vi "Main_old.vi"() -> ()   [LabVIEW 2021]
uses:
  TypeDefs/DevInfo.ctl
  TypeDefs/TargetAccess.ctl
  <vilib>/nisyscfg/Network Settings Format.ctl
  <userlib>/S2 Labs/Error Reporting/Transport_WinDebug/Transport_WinDebug.lvclass
  C:/Program Files (x86)/National Instruments/LabVIEW 2021/user.lib/S2 Labs/Error Reporting/Transport Class/Transport.lvclass
  <vilib>/nisyscfg/Close (System).vi
  <vilib>/nisyscfg/Format 5.3.vi
  <vilib>/nisyscfg/Save Changes (Hardware).vi
  <vilib>/nisyscfg/Close (Hardware).vi
  <vilib>/nisyscfg/Save Changes (System).vi
  <vilib>/nisyscfg/nisyscfg.lvlib
  <resource>/objmgr/nisysapi.rc
  <userlib>/S2 Labs/Error Reporting/Error Reporting.lvlib
  <resource>/objmgr/nicontrollersysapi.rc
panel:
  in  "Abort":bool
  out "n":i32
  out "of":i32
  out "Refreshing":bool
  in  "Device List":i32(listbox)
  out "MAC":string
  out "OS":string
  out "Firmware":string
  out "Status":string
  out "Version":string
  out "Description":string
  out "Title":string
  out "Model":string
  in  "ChangePassword":bool
  in  "ChangeMode":bool
  in  "Restart":bool
  in  "FormatDisk":bool
  in  "ManageFeeds":bool
  in  "DeplyFW":bool
  in  "NetworkSettings":bool
  in  "Refresh":bool
  in  "DeplyImg":bool
  in  "RetrieveImg":bool
  # "Device Properties"
  # "Image Properties"
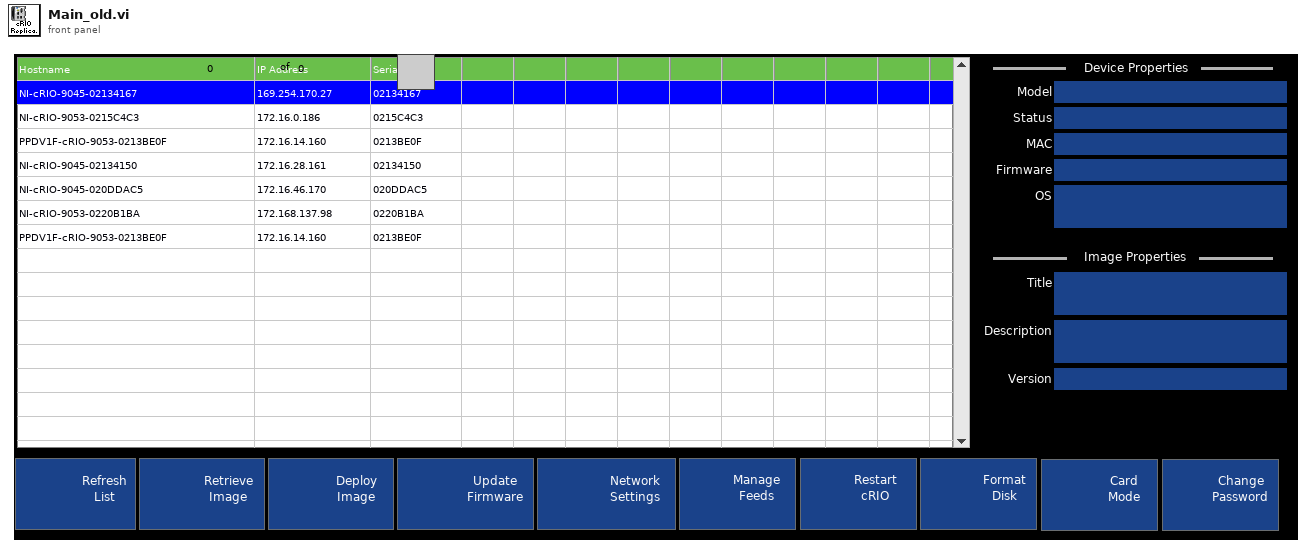
[diagram p1: front panel]
types:
  T1 = typedef "DevInfo.ctl" = cluster{"Hostname":string, "IPAddress":string, "MAC":string, "SerialNum":string, "Model":string, "Status":string, "FW":string, "OSDesc":string, "ImgTitle":string, "ImgDesc":string, "ImgVer":string, "ImgID":string, "IP Address Request Mode":i32, "SubnetMask":string, "Gateway":string, "DNSServer":string}
  T2 = enum8{"Enabled", "Disabled", "Disabled and Grayed Out"}
  T3 = typedef "TargetAccess.ctl" = enum16{"Read-Only", "Admin"}
  T4 = typedef "nisyscfg.lvlib/Network Settings Format.ctl" = u32
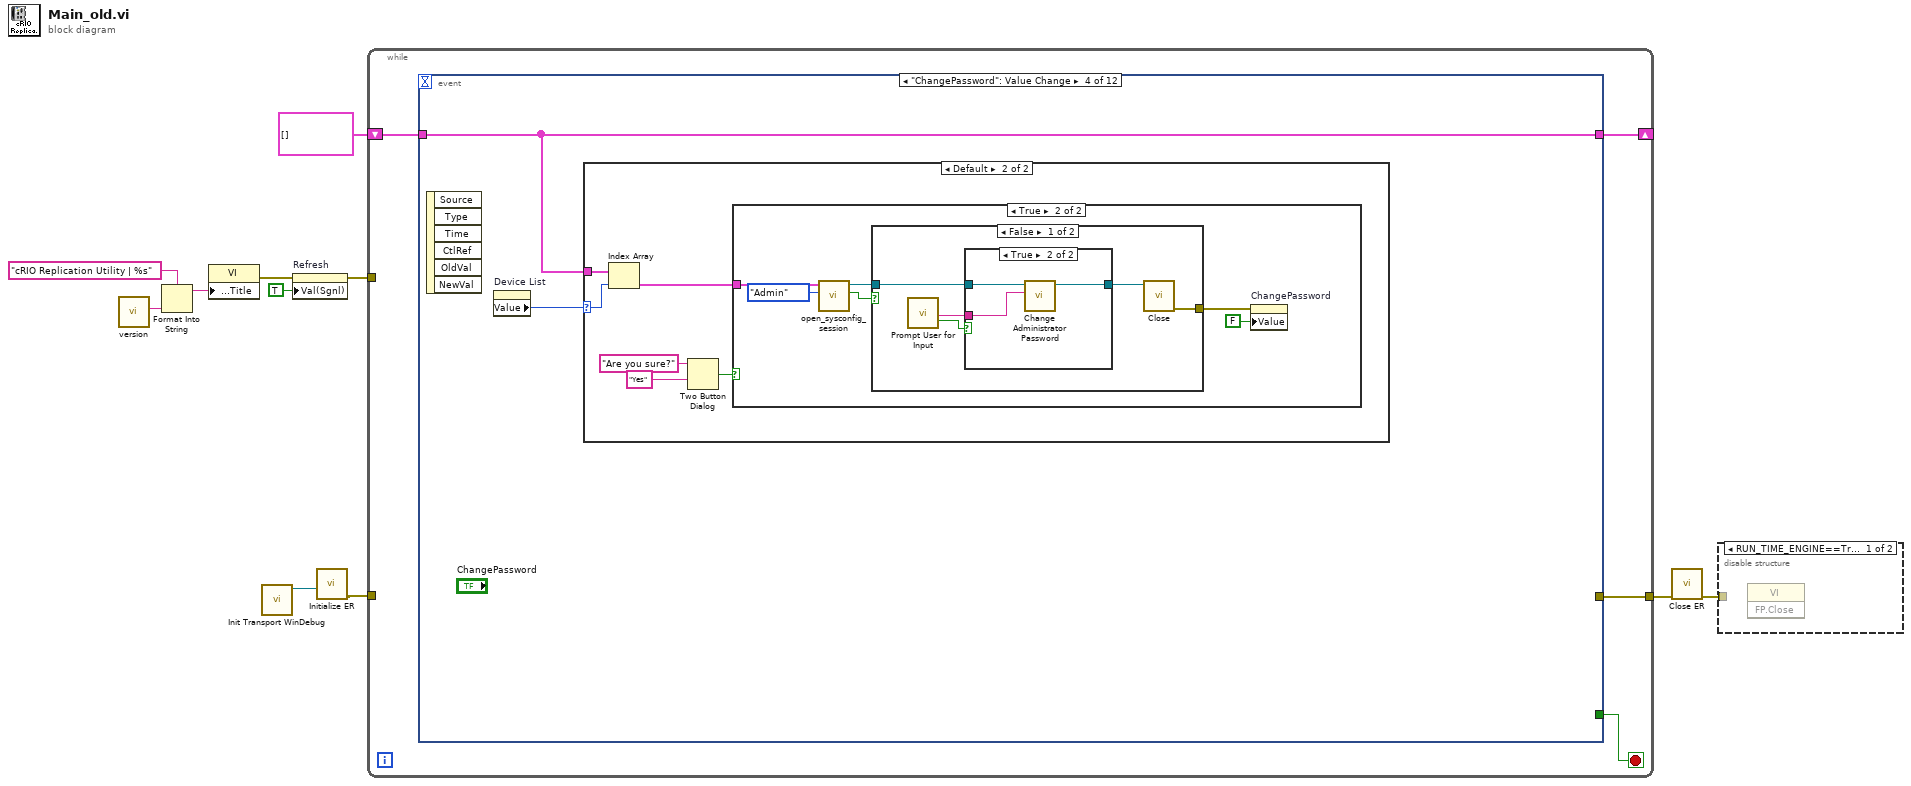
[diagram p0: block diagram]
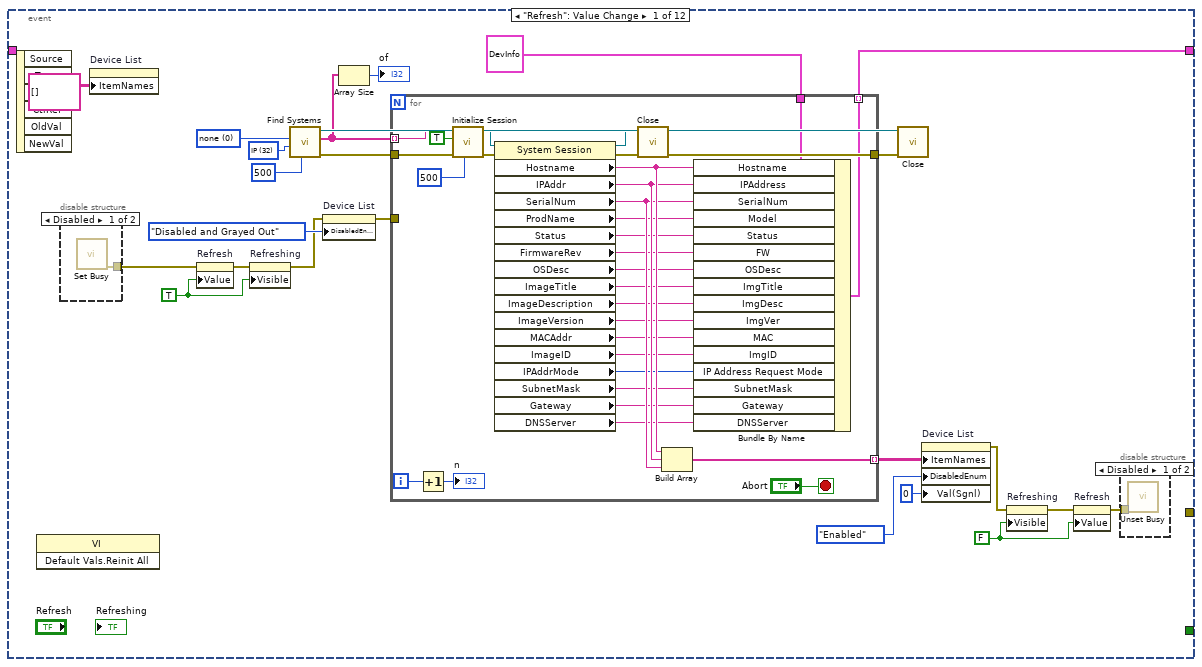
[diagram p3: hidden frame]
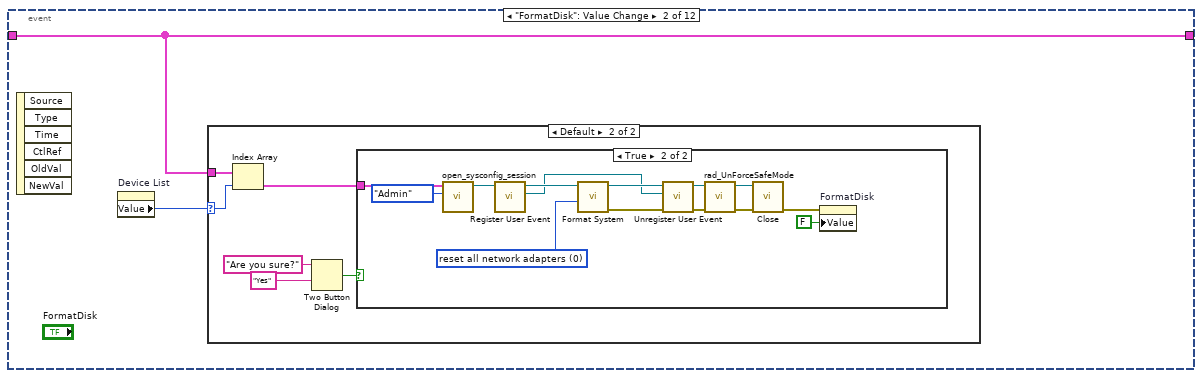
[diagram p6: hidden frame]
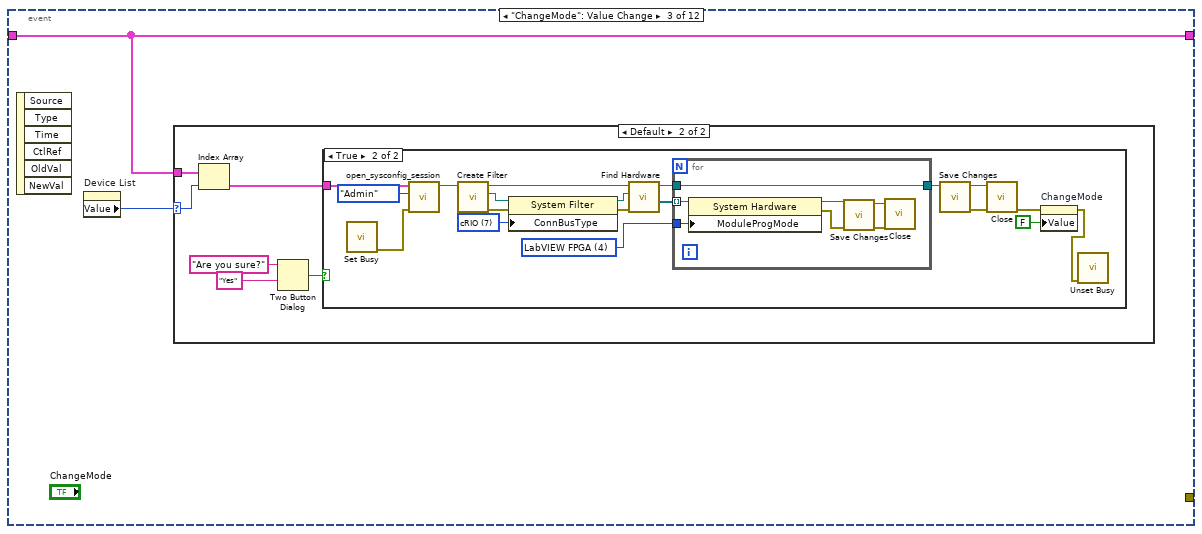
[diagram p9: hidden frame]
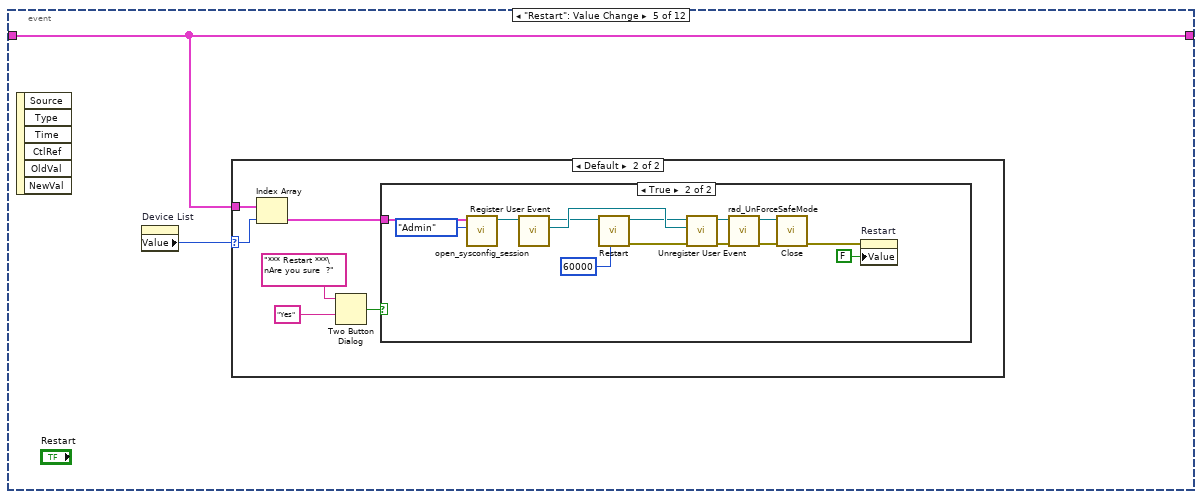
[diagram p16: hidden frame]
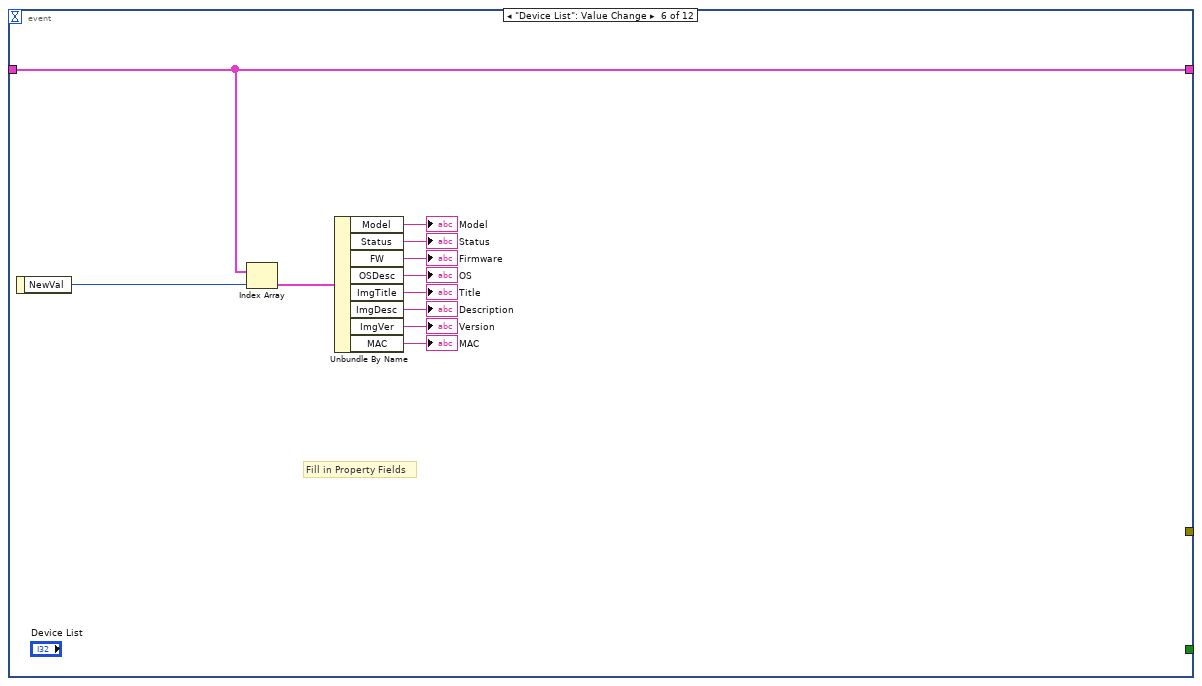
[diagram p19: hidden frame]
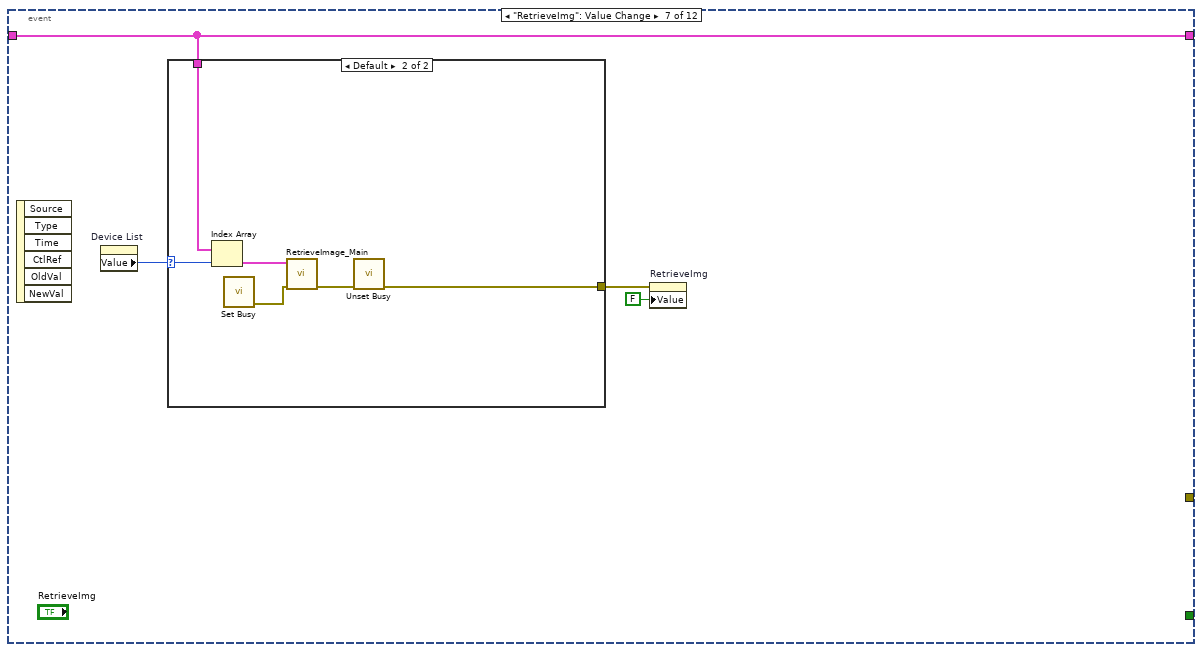
[diagram p20: hidden frame]
diagram:
  n1 = call "version.vi"() -> ("version"=w5:string)  [unwired: 11 in]
  n2 = Format Into String(format string="cRIO Replication Utility | %s", w5) -> (resulting string=w4:string)  [unwired: 2 in, 1 out]
  n3 = property class="VI"("Front Panel.Title"=w4) -> (error out=w3:errorcluster)  [unwired: 2 in, 1 out]
  n4 = call <userlib>:"Init Transport WinDebug.vi"() -> ("Transport WinDebug"=w8:refnum<class "Transport_WinDebug.lvclass">)  [unwired: 11 in]
  n5 = property on="Refresh" class="Bool (strict)"(error in=w3, "Val(Sgnl)"=TRUE ("Value (Signaling)")) -> (error out=w2:errorcluster)  [unwired: 1 in, 1 out]
  n6 = call <userlib>:"Initialize ER.vi"("Transport Class (UDP)"=w8) -> ("error out"=w9:errorcluster)  [unwired: 10 in]
  n7 = while {
    shift-right: [w13] -> _
    shift-left: T1[] [] -> [w14]
    tunnel: w9 -> [_]
    tunnel: [w12] -> w7
    tunnel: w2 -> [_]
    stop <- w15 stop-if-true
    n8 = event shown="[3] \"ChangePassword\": Value Change" {
      selector: _ -> [_ _ _ _ _ _ _ _ _ _ _ _]
      dyn-events: _ -> [_ _ _ _ _ _ _ _ _ _ _ _]
      timeout: _ -> [_ _ _ _ _ _ _ _ _ _ _ _]
      tunnel: [_ _ _ _ _ _ _ _ _ _ _ TRUE] -> w15
      tunnel: w14 -> [_ w73 w95 w129 w152 w184 w187 w197 w207 w217 w227 w236]
      tunnel: [w19 w73 w95 w129 w152 w184 w187 w197 w207 w217 w227 w236] -> w13
      tunnel: [_ _ _ _ _ _ _ _ _ _ _ errorcluster {"status"=FALSE, "code"=0, "source"=""} ("error out")] -> w12
      event "Refresh": Value Change {
        w25 = FALSE ("Visible")
        w26 = TRUE ("Visible")
        w36 = u32 0 items=["none"=0, "only if online"=1, "all"=3] ("Include Cached Results (all)")
        w39 = u32 32 items=["Hostname"=16, "Hostname (IP)"=18, "Hostname (MAC)"=19, "IP"=32, "IP (Hostname)"=33, "IP (MAC)"=35, "MAC"=48, "MAC (Hostname)"=49, "MAC (IP)"=50] ("Output (Hostname and IP)")
        n9 = event-data() -> ()  [unwired: 1 in, 6 out]
        n10 = invoke class="VI" method="Default Vals.Reinit All"() -> ()  [unwired: 3 in, 3 out]
        n11 = disable-structure shown="Disabled" {
          disable-tunnel: [w41 _] -> w23
          frame Disabled {
            n12 = call <vilib>:"Set Busy.vi"() -> ("error out"=w41:errorcluster)  [unwired: 10 in, 1 out]
          }
          frame Enabled {
          }
        }
        n13 = property on="Device List" class="MCListbox (strict)"("ItemNames"=string[][] [] ("Item Names")) -> ()  [unwired: 2 in, 2 out]
        n14 = property on="Refresh" class="Bool (strict)"(error in=w23, "Value"=w26) -> (error out=w27:errorcluster)  [unwired: 1 in, 1 out]
        n15 = property on="Refreshing" class="Bool (strict)"(error in=w27, "Visible"=w26) -> (error out=w29:errorcluster)  [unwired: 1 in, 1 out]
        n16 = call <vilib>:"Find Systems.vi"("Timeout (4000 ms)"=u32 500, "Output (Hostname and IP)"=w39, "Include Cached Results (all)"=w36) -> ("error out"=w33:errorcluster, "Detected Systems"=w17:string[], "Session out"=w37:refnum<k21>)  [unwired: 6 in]
        n17 = property on="Device List" class="MCListbox (strict)"(error in=w29, "DisabledEnum"=T2."Disabled and Grayed Out" ("Disabled")) -> (error out=w31:errorcluster)  [unwired: 1 in, 1 out]
        n18 = Array Size(array=w17) -> (size(s)=→"of":i32)
        n19 = for {
          tunnel: w17 -> [w71] mode=indexing
          tunnel: [w70] -> w34 mode=indexing
          tunnel: [w68] -> w38
          tunnel: w33 -> [w64]
          tunnel: w31 -> [_]
          tunnel: T1 {"Hostname"="", "IPAddress"="", "MAC"="", "SerialNum"="", "Model"="", "Status"="", "FW"="", "OSDesc"="", "ImgTitle"="", "ImgDesc"="", "ImgVer"="", "ImgID"="", "IP Address Request Mode"=1, "SubnetMask"="", "Gateway"="", "DNSServer"=""} ("DevInfo") -> [w62]
          tunnel: [w52] -> w19 mode=indexing
          i -> [w44]
          stop <- "Abort" stop-if-true
          n20 = Increment(x=w44) -> (x+1=→"n":i32)
          n21 = call <vilib>:"Initialize Session.vi"("Connect Timeout (4000 ms)"=u32 500, "error in (no error)"=w64, "Force Property Refresh (T)"=TRUE, "Target (localhost)"=w71) -> ("error out"=w66:errorcluster, "Session out"=w72:refnum<k21>)  [unwired: 6 in]
          n22 = property class="System Session"(reference=w72, error in=w66) -> (reference out=w69:refnum<k21>, error out=w65:errorcluster, "Hostname"=w61:string, "IPAddr"=w60:string, "SerialNum"=w59:string, "ProdName"=w51:string, "Status"=w58:string, "FirmwareRev"=w57:string, "OSDesc"=w56:string, "ImageTitle"=w55:string, "ImageDescription"=w54:string, "ImageVersion"=w53:string, "MACAddr"=w50:string, "ImageID"=w49:string, "IPAddrMode"=w48:i32, "SubnetMask"=w47:string, "Gateway"=w46:string, "DNSServer"=w45:string)
          n23 = call-poly <vilib>:"Close.vi"("error in (no error)"=w65, "Session in"=w69) -> ("error out"=w68:errorcluster)  [unwired: 9 in]
          n24 = Build Array(w61, w60, w59) -> (w70:string[])
          n25 = Bundle By Name(cluster=w62, "Hostname"=w61, "IPAddress"=w60, "SerialNum"=w59, "Model"=w51, "Status"=w58, "FW"=w57, "OSDesc"=w56, "ImgTitle"=w55, "ImgDesc"=w54, "ImgVer"=w53, "MAC"=w50, "ImgID"=w49, "IP Address Request Mode"=w48, "SubnetMask"=w47, "Gateway"=w46, "DNSServer"=w45) -> (w52:T1)
        }
        n26 = call-poly <vilib>:"Close.vi"("error in (no error)"=w38, "Session in"=w37) -> ()  [unwired: 9 in, 1 out]
        n27 = property on="Device List" class="MCListbox (strict)"("ItemNames"=w34, "DisabledEnum"=T2."Enabled" ("Disabled"), "Val(Sgnl)"=0 ("Value (Signaling)")) -> (error out=w28:errorcluster)  [unwired: 2 in, 1 out]
        n28 = property on="Refreshing" class="Bool (strict)"(error in=w28, "Visible"=w25) -> (error out=w24:errorcluster)  [unwired: 1 in, 1 out]
        n29 = property on="Refresh" class="Bool (strict)"(error in=w24, "Value"=w25) -> (error out=w22:errorcluster)  [unwired: 1 in, 1 out]
        n30 = disable-structure shown="Disabled" {
          disable-tunnel: w22 -> [w40 _]
          frame Disabled {
            n31 = call <vilib>:"Unset Busy.vi"("error in (no error)"=w40) -> ()  [unwired: 10 in, 1 out]
          }
          frame Enabled {
          }
        }
      }
      event "FormatDisk": Value Change {
        n32 = event-data() -> ()  [unwired: 1 in, 6 out]
        n33 = property on="Device List" class="MCListbox (strict)"() -> ("Value"=w74:i32)  [unwired: 2 in, 2 out]
        n34 = case shown="Default" w74 {
          selector: w74 -> [_ w79]
          tunnel: w73 -> [_ w80]
          frame -1 {
          }
          frame Default {
            n35 = Index Array(array=w80, index=w79) -> (element=w75:T1)
            n36 = Two Button Dialog(message="Are you sure?", 2:"Yes" ("T button name (\"OK\")")) -> (T button?=w76:bool)  [unwired: 1 in]
            n37 = case shown="True" w76 {
              tunnel: w75 -> [_ w92]
              frame False {
              }
              frame True {
                w91 = T4 0 items=["reset all network adapters", "preserve primary, reset others", "preserve all network adapters"] ("Network Settings (reset all adapters)")
                n38 = call "open_sysconfig_session.vi"("Target Access"=TargetAccess."Admin", "DevInfo"=w92) -> ("Session Out"=w93:refnum<k21>)  [unwired: 7 in, 2 out]
                n39 = call <vilib>:"Register User Event.vi"("Session in"=w93) -> ("Event Registration out"=w83:refnum<event-registration>, "Session out"=w90:refnum<k21>)  [unwired: 8 in, 1 out]
                n40 = call-poly <vilib>:"Format System.vi"("Network Settings (reset all adapters)"=w91, "Session in"=w90) -> ("error out"=w87:errorcluster, "Session out"=w86:refnum<k21>)  [unwired: 8 in]
                n41 = call <vilib>:"Unregister User Event.vi"("error in (no error)"=w87, "Event Registration in"=w83, "Session in"=w86) -> ("error out"=w88:errorcluster, "Session out"=w89:refnum<k21>)  [unwired: 7 in]
                n42 = call "rad_UnForceSafeMode.vi"("error in (no error)"=w88, "Target in"=w89) -> ("error out"=w84:errorcluster, "Target out"=w85:refnum<k21>)  [unwired: 8 in]
                n43 = call-poly <vilib>:"Close.vi"("error in (no error)"=w84, "Session in"=w85) -> ("error out"=w82:errorcluster)  [unwired: 9 in]
                n44 = property on="FormatDisk" class="Bool (strict)"(error in=w82, "Value"=FALSE ("FormatDisk")) -> ()  [unwired: 1 in, 2 out]
              }
            }
          }
        }
      }
      event "ChangeMode": Value Change {
        n45 = event-data() -> ()  [unwired: 1 in, 6 out]
        n46 = property on="Device List" class="MCListbox (strict)"() -> ("Value"=w96:i32)  [unwired: 2 in, 2 out]
        n47 = case shown="Default" w96 {
          selector: w96 -> [_ w101]
          tunnel: w95 -> [_ w102]
          frame -1 {
          }
          frame Default {
            n48 = Index Array(array=w102, index=w101) -> (element=w97:T1)
            n49 = Two Button Dialog(message="Are you sure?", 2:"Yes" ("T button name (\"OK\")")) -> (T button?=w98:bool)  [unwired: 1 in]
            n50 = case shown="True" w98 {
              tunnel: w97 -> [_ w120]
              frame False {
              }
              frame True {
                w108 = u32 4 items=["None"=0, "Real-Time CPU"=1, "Real-Time Scan Engine"=2, "LabVIEW FPGA"=4] ("Devices & Chassis:Bus Specific:cRIO Module Programming Mode")
                w107 = u32 7 items=["BuiltIn/System", "PXI/PCI", "USB", "GPIB", "VXI", "Serial", "TCP/IP", "cRIO", "SCXI", "cDAQ", "SwitchBlock", "SCC", "FireWire", "Accessory", "CAN", "SwitchBlock Device", "SLSC"] ("Devices & Chassis:Connects To Bus Type")
                n51 = call <vilib>:"Set Busy.vi"() -> ("error out"=w104:errorcluster)  [unwired: 10 in, 1 out]
                n52 = call "open_sysconfig_session.vi"("error in (no error)"=w104, "Target Access"=TargetAccess."Admin", "DevInfo"=w120) -> ("Session Out"=w106:refnum<k21>)  [unwired: 6 in, 2 out]
                n53 = call <vilib>:"Create Filter.vi"("Session in"=w106) -> ("error out"=w109:errorcluster, "Filter out"=w110:refnum<k20>, "Session out"=w113:refnum<k21>)  [unwired: 8 in]
                n54 = property class="System Filter"(reference=w110, error in=w109, "ConnBusType"=w107) -> (reference out=w112:refnum<k20>, error out=w111:errorcluster)
                n55 = call <vilib>:"Find Hardware.vi"("error in (no error)"=w111, "Filter in"=w112, "Session in"=w113) -> ("Resources out"=w114:refnum<k20>[], "Session out"=w115:refnum<k21>)  [unwired: 5 in, 2 out]
                n56 = for {
                  tunnel: w114 -> [w128] mode=indexing
                  tunnel: w115 -> [w123]
                  tunnel: [w123] -> w116
                  tunnel: w108 -> [w122]
                  n57 = property class="System Hardware"(reference=w128, "ModuleProgMode"=w122) -> (reference out=w125:refnum<k20>, error out=w127:errorcluster)  [unwired: 1 in]
                  n58 = call-poly <vilib>:"Save Changes.vi"("error in (no error)"=w127, "Resource in"=w125) -> ("error out"=w124:errorcluster, "Resource out"=w126:refnum<k20>)  [unwired: 6 in, 2 out]
                  n59 = call-poly <vilib>:"Close.vi"("error in (no error)"=w124, "Resource in"=w126) -> ()  [unwired: 9 in, 1 out]
                }
                n60 = call-poly <vilib>:"Save Changes.vi"("Session in"=w116) -> ("error out"=w118:errorcluster, "Session out"=w117:refnum<k21>)  [unwired: 7 in, 2 out]
                n61 = call-poly <vilib>:"Close.vi"("error in (no error)"=w118, "Session in"=w117) -> ("error out"=w105:errorcluster)  [unwired: 9 in]
                n62 = property on="ChangeMode" class="Bool (strict)"(error in=w105, "Value"=FALSE ("FormatDisk")) -> (error out=w103:errorcluster)  [unwired: 1 in, 1 out]
                n63 = call <vilib>:"Unset Busy.vi"("error in (no error)"=w103) -> ()  [unwired: 10 in, 1 out]
              }
            }
          }
        }
      }
      event "ChangePassword": Value Change {
        n64 = event-data() -> ()  [unwired: 1 in, 6 out]
        n65 = property on="Device List" class="MCListbox (strict)"() -> ("Value"=w130:i32)  [unwired: 2 in, 2 out]
        n66 = case shown="Default" w130 {
          selector: w130 -> [_ w135]
          tunnel: w129 -> [_ w136]
          frame -1 {
          }
          frame Default {
            n67 = Index Array(array=w136, index=w135) -> (element=w131:T1)
            n68 = Two Button Dialog(message="Are you sure?", 2:"Yes" ("T button name (\"OK\")")) -> (T button?=w132:bool)  [unwired: 1 in]
            n69 = case shown="True" w132 {
              tunnel: w131 -> [_ w141]
              frame False {
              }
              frame True {
                n70 = call "open_sysconfig_session.vi"("Target Access"=TargetAccess."Admin", "DevInfo"=w141) -> ("Cancelled"=w137:bool, "Session Out"=w138:refnum<k21>)  [unwired: 7 in, 1 out]
                n71 = case shown="False" w137 {
                  tunnel: [w147 _] -> w139
                  tunnel: w138 -> [w146 _]
                  frame False {
                    n72 = call "Prompt User for Input"() -> ("New Password"=w144:string, "OK"=w143:bool)  [unwired: 17 in, 1 out]
                    n73 = case shown="True" w143 {
                      tunnel: w146 -> [w148 w151]
                      tunnel: [w148 w150] -> w145
                      tunnel: w144 -> [_ w149]
                      frame False {
                      }
                      frame True {
                        n74 = call <vilib>:"Change Administrator Password.vi"("New Password"=w149, "Session in"=w151) -> ("Session out"=w150:refnum<k21>)  [unwired: 8 in, 1 out]
                      }
                    }
                    n75 = call-poly <vilib>:"Close.vi"("Session in"=w145) -> ("error out"=w147:errorcluster)  [unwired: 10 in]
                  }
                  frame True {
                  }
                }
                n76 = property on="ChangePassword" class="Bool (strict)"(error in=w139, "Value"=FALSE ("FormatDisk")) -> ()  [unwired: 1 in, 2 out]
              }
            }
          }
        }
      }
      event "Restart": Value Change {
        n77 = event-data() -> ()  [unwired: 1 in, 6 out]
        n78 = property on="Device List" class="MCListbox (strict)"() -> ("Value"=w153:i32)  [unwired: 2 in, 2 out]
        n79 = case shown="Default" w153 {
          selector: w153 -> [_ w158]
          tunnel: w152 -> [_ w159]
          frame -1 {
          }
          frame Default {
            n80 = Index Array(array=w159, index=w158) -> (element=w154:T1)
            n81 = Two Button Dialog(message="*** Restart ***\nAre you sure  ?", 2:"Yes" ("T button name (\"OK\")")) -> (T button?=w155:bool)  [unwired: 1 in]
            n82 = case shown="True" w155 {
              tunnel: w154 -> [_ w171]
              frame False {
              }
              frame True {
                n83 = call "open_sysconfig_session.vi"("Target Access"=TargetAccess."Admin", "DevInfo"=w171) -> ("Session Out"=w172:refnum<k21>)  [unwired: 7 in, 2 out]
                n84 = call <vilib>:"Register User Event.vi"("Session in"=w172) -> ("Event Registration out"=w166:refnum<event-registration>, "Session out"=w165:refnum<k21>)  [unwired: 8 in, 1 out]
                n85 = call <vilib>:"Restart.vi"("Timeout (180,000 ms)"=u32 60000, "Session in"=w165) -> ("error out"=w163:errorcluster, "Session out"=w164:refnum<k21>)  [unwired: 7 in, 1 out]
                n86 = call <vilib>:"Unregister User Event.vi"("error in (no error)"=w163, "Event Registration in"=w166, "Session in"=w164) -> ("error out"=w169:errorcluster, "Session out"=w170:refnum<k21>)  [unwired: 7 in]
                n87 = call "rad_UnForceSafeMode.vi"("error in (no error)"=w169, "Target in"=w170) -> ("error out"=w167:errorcluster, "Target out"=w168:refnum<k21>)  [unwired: 8 in]
                n88 = call-poly <vilib>:"Close.vi"("error in (no error)"=w167, "Session in"=w168) -> ("error out"=w160:errorcluster)  [unwired: 9 in]
                n89 = property on="Restart" class="Bool (strict)"(error in=w160, "Value"=FALSE ("Restart")) -> ()  [unwired: 1 in, 2 out]
              }
            }
          }
        }
      }
      event "Device List": Value Change {
        # "Fill in Property Fields"
        n90 = event-data() -> ("NewVal"=w183:i32)  [unwired: 1 in]
        n91 = Index Array(array=w184, index=w183) -> (element=w182:T1)
        n92 = Unbundle By Name(w182) -> ("Model"=→"Model":string, "Status"=→"Status":string, "FW"=→"Firmware":string, "OSDesc"=→"OS":string, "ImgTitle"=→"Title":string, "ImgDesc"=→"Description":string, "ImgVer"=→"Version":string, "MAC"=→"MAC":string)
      }
      event "RetrieveImg": Value Change {
        n93 = event-data() -> ()  [unwired: 1 in, 6 out]
        n94 = property on="Device List" class="MCListbox (strict)"() -> ("Value"=w188:i32)  [unwired: 2 in, 2 out]
        n95 = case shown="Default" w188 {
          selector: w188 -> [_ w193]
          tunnel: w187 -> [_ w194]
          tunnel: [_ w189] -> w185
          frame -1 {
          }
          frame Default {
            n96 = Index Array(array=w194, index=w193) -> (element=w192:T1)
            n97 = call <vilib>:"Set Busy.vi"() -> ("error out"=w191:errorcluster)  [unwired: 10 in, 1 out]
            n98 = call "RetrieveImage_Main.vi"("error in (no error)"=w191, "DevInfo"=w192) -> ("error out"=w190:errorcluster)  [unwired: 9 in]
            n99 = call <vilib>:"Unset Busy.vi"("error in (no error)"=w190) -> ("error out"=w189:errorcluster)  [unwired: 10 in]
          }
        }
        n100 = property on="RetrieveImg" class="Bool (strict)"(error in=w185, "Value"=FALSE ("RetrieveImg")) -> ()  [unwired: 1 in, 2 out]
      }
      event "DeplyImg": Value Change {
        n101 = event-data() -> ()  [unwired: 1 in, 6 out]
        n102 = property on="Device List" class="MCListbox (strict)"() -> ("Value"=w198:i32)  [unwired: 2 in, 2 out]
        n103 = case shown="Default" w198 {
          selector: w198 -> [_ w203]
          tunnel: w197 -> [_ w204]
          tunnel: [_ w199] -> w195
          frame -1 {
          }
          frame Default {
            n104 = Index Array(array=w204, index=w203) -> (element=w202:T1)
            n105 = call <vilib>:"Set Busy.vi"() -> ("error out"=w201:errorcluster)  [unwired: 10 in, 1 out]
            n106 = call "DeployImage_Main.vi"("error in (no error)"=w201, "DevInfo"=w202) -> ("error out"=w200:errorcluster)  [unwired: 9 in]
            n107 = call <vilib>:"Unset Busy.vi"("error in (no error)"=w200) -> ("error out"=w199:errorcluster)  [unwired: 10 in]
          }
        }
        n108 = property on="DeplyImg" class="Bool (strict)"(error in=w195, "Value"=FALSE ("DeplyImg")) -> ()  [unwired: 1 in, 2 out]
      }
      event "DeplyFW": Value Change {
        n109 = event-data() -> ()  [unwired: 1 in, 6 out]
        n110 = property on="Device List" class="MCListbox (strict)"() -> ("Value"=w208:i32)  [unwired: 2 in, 2 out]
        n111 = case shown="Default" w208 {
          selector: w208 -> [_ w213]
          tunnel: w207 -> [_ w214]
          tunnel: [_ w212] -> w205
          frame -1 {
          }
          frame Default {
            n112 = Index Array(array=w214, index=w213) -> (element=w209:T1)
            n113 = call <vilib>:"Set Busy.vi"() -> ("error out"=w211:errorcluster)  [unwired: 10 in, 1 out]
            n114 = call "UpgradeFirmware_Main.vi"("error in (no error)"=w211, "DevInfo"=w209) -> ("error out"=w210:errorcluster)  [unwired: 9 in]
            n115 = call <vilib>:"Unset Busy.vi"("error in (no error)"=w210) -> ("error out"=w212:errorcluster)  [unwired: 10 in]
          }
        }
        n116 = property on="DeplyFW" class="Bool (strict)"(error in=w205, "Value"=FALSE ("DeplyImg")) -> ()  [unwired: 1 in, 2 out]
      }
      event "ManageFeeds": Value Change {
        n117 = event-data() -> ()  [unwired: 1 in, 6 out]
        n118 = property on="Device List" class="MCListbox (strict)"() -> ("Value"=w218:i32)  [unwired: 2 in, 2 out]
        n119 = case shown="Default" w218 {
          selector: w218 -> [_ w221]
          tunnel: w217 -> [_ w222]
          tunnel: [_ w219] -> w215
          frame -1 {
          }
          frame Default {
            n120 = Index Array(array=w222, index=w221) -> (element=w220:T1)
            n121 = call "Feed_Main.vi"("DevInfo"=w220) -> ("error out"=w219:errorcluster)  [unwired: 10 in]
          }
        }
        n122 = property on="ManageFeeds" class="Bool (strict)"(error in=w215, "Value"=FALSE ("ManageFeeds")) -> ()  [unwired: 1 in, 2 out]
      }
      event "NetworkSettings": Value Change {
        n123 = event-data() -> ()  [unwired: 1 in, 6 out]
        n124 = property on="Device List" class="MCListbox (strict)"() -> ("Value"=w228:i32)  [unwired: 2 in, 2 out]
        n125 = case shown="Default" w228 {
          selector: w228 -> [_ w233]
          tunnel: w227 -> [_ w234]
          tunnel: [_ w231] -> w223
          tunnel: [_ w230] -> w226
          frame -1 {
          }
          frame Default {
            n126 = Index Array(array=w234, index=w233) -> (element=w232:T1)
            n127 = call "Network_Main.vi"("DevInfo"=w232) -> ("error out"=w231:errorcluster, "Cancelled"=w230:bool)  [unwired: 9 in]
          }
        }
        n128 = Or(x=w226, y=w223) -> (x .or. y?=w224:bool)
        n129 = property on="NetworkSettings" class="Bool (strict)"(error in=w223, "Value"=FALSE ("DeplyImg")) -> ()  [unwired: 1 in, 2 out]
        n130 = case shown="False" w224 {
          frame False {
            n131 = property on="Refresh" class="Bool (strict)"("Val(Sgnl)"=TRUE ("Value (Signaling)")) -> ()  [unwired: 2 in, 2 out]
          }
          frame True {
          }
        }
      }
      event Panel Close? {
        n132 = event-data() -> ()  [unwired: 1 in, 4 out]
        n133 = event-data("Discard?"=TRUE) -> ()  [unwired: 1 in, 1 out]
      }
    }
  }
  n134 = call <userlib>:"Close ER.vi"("error in (no error)"=w7) -> ("error out"=w1:errorcluster)  [unwired: 10 in]
  n135 = disable-structure shown="RUN_TIME_ENGINE==True" {
    disable-tunnel: w1 -> [_ _]
    frame condition #0 {
      n136 = invoke class="VI" method="FP.Close"() -> ()  [unwired: 3 in, 3 out]
    }
    frame condition #1 (active) {
    }
  }
